vi "jMsg_SnakeProcessor_AddPlayer - Rx Read.vi"(8 "error in (no error)":errorcluster, 11 "jModule":refnum<class "jModule.lvclass">) -> (0 "error out":errorcluster, 2 "Player":refnum<class "Player.lvclass">, 3 "jModule":refnum<class "jModule.lvclass">, 7 "jMsg_SnakeProcessor_AddPlayer":refnum<class "jMsg_SnakeProcessor_AddPlayer.lvclass">)   [LabVIEW 2019, in "jMsg_SnakeProcessor_AddPlayer.lvclass"]
doc: "This VI is used to read data from the jMsg\n\n\nJSMA Message Wizard 0.2.0.5\nRob Humfeld - Jet Engineering\nCopyright (c) 2020, Jet Engineering"
uses:
  jMsg_SnakeProcessor_AddPlayer.lvclass
  <userlib>/Jet Engineering/JSMA/Libraries/jModule Class/jModule.lvclass
  Player/Player.lvclass
  <userlib>/Jet Engineering/JSMA/Libraries/jModule Class/jModule.lvclass/jModule.ctl
  jMsg_SnakeProcessor_AddPlayer.lvclass/jMsg_SnakeProcessor_AddPlayer.ctl
panel:
  in  "jMsg_SnakeProcessor_AddPlayer":refnum<class "jMsg_SnakeProcessor_AddPlayer.lvclass">
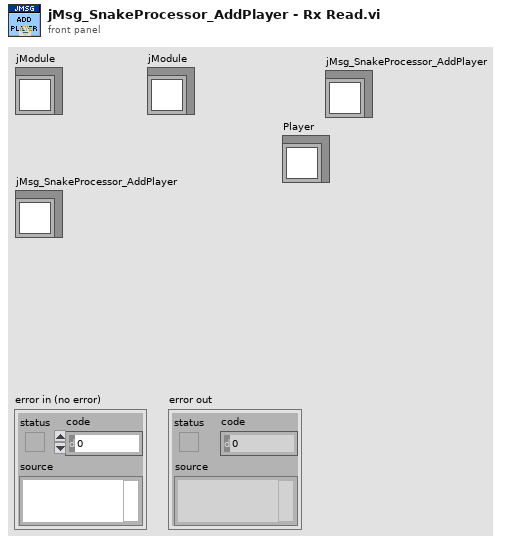
[diagram p1: front panel]
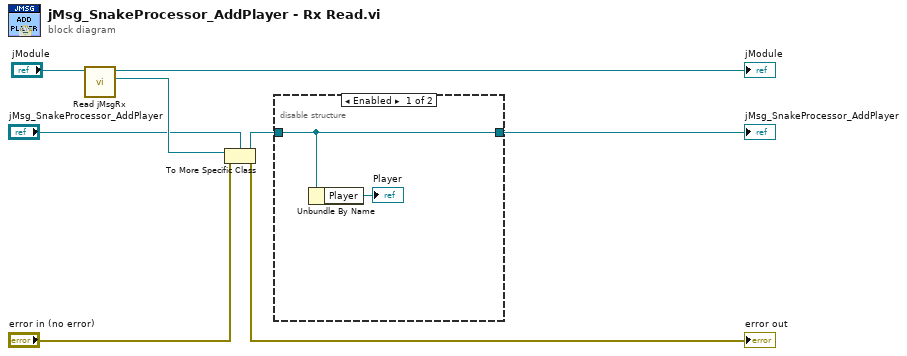
[diagram p0: block diagram]
diagram:
  n1 = call <userlib>:"Read jMsgRx.vi"("jModule in"="jModule") -> ("Received jMsg"=w5:refnum<class "jMsg.lvclass">, "jModule out"=→"jModule":refnum<class "jModule.lvclass">)  [unwired: 8 in, 1 out]
  n2 = To More Specific Class(target class="jMsg_SnakeProcessor_AddPlayer", reference=w5, error in="error in (no error)") -> (specific class reference=w3:refnum<class "jMsg_SnakeProcessor_AddPlayer.lvclass">, error out=→"error out":errorcluster)
  n3 = disable-structure shown="Enabled" {
    disable-tunnel: w3 -> [w10 w11]
    disable-tunnel: [w10 w11] -> w8
    frame Enabled {
      n4 = Unbundle By Name(w10) -> ("Player"=→"Player":refnum<class "Player.lvclass">)
    }
    frame Disabled {
    }
  }
  "jMsg_SnakeProcessor_AddPlayer" <- w8
